vi "Test Path 1.vi"() -> (4 "path":cluster{"X":dbl, "Y":dbl}[](array[cluster])=[{"X"=67.5, "Y"=162.0}, {"X"=149.75257731958763, "Y"=161.43554006968643}, {"X"=169.7938144329897, "Y"=66.60627177700349}, {"X"=262.2061855670103, "Y"=62.09059233449478}, {"X"=279.4639175257732, "Y"=97.65156794425087}, {"X"=279.4639175257732, "Y"=115.14982578397213}])   [LabVIEW 2018]
uses:
  AutonBuilder/Typedef/Data Point.ctl
panel:
  in  "Data Points":T1[](array[typedef])=[{"X"=67.5, "Y"=162.0, "Theta"=0.0, "Speed %"=0.0, "Disabled?"=FALSE}, {"X"=149.75257731958763, "Y"=161.43554006968643, "Theta"=0.0, "Speed %"=0.0, "Disabled?"=FALSE}, {"X"=169.7938144329897, "Y"=66.60627177700349, "Theta"=0.0, "Speed %"=0.0, "Disabled?"=FALSE}, {"X"=262.2061855670103, "Y"=62.09059233449478, "Theta"=0.0, "Speed %"=0.0, "Disabled?"=FALSE}, {"X"=279.4639175257732, "Y"=97.65156794425087, "Theta"=0.0, "Speed %"=0.0, "Disabled?"=FALSE}, {"X"=279.4639175257732, "Y"=115.14982578397213, "Theta"=0.0, "Speed %"=0.0, "Disabled?"=FALSE}]
  out "Graph":cluster{dbl[], dbl[]}[](graph)=[{[48.0, 81.5, 81.5, 48.0, 48.0], [176.25, 176.25, 147.75, 147.75, 176.25]}, {[67.5, 149.75257731958763, 169.7938144329897, 262.2061855670103, 279.4639175257732, 279.4639175257732], [162.0, 161.43554006968643, 66.60627177700349, 62.09059233449478, 97.65156794425087, 115.14982578397213]}, {array[332 elements], array[332 elements]}, {array[332 elements], array[332 elements]}, {array[332 elements], array[332 elements]}]
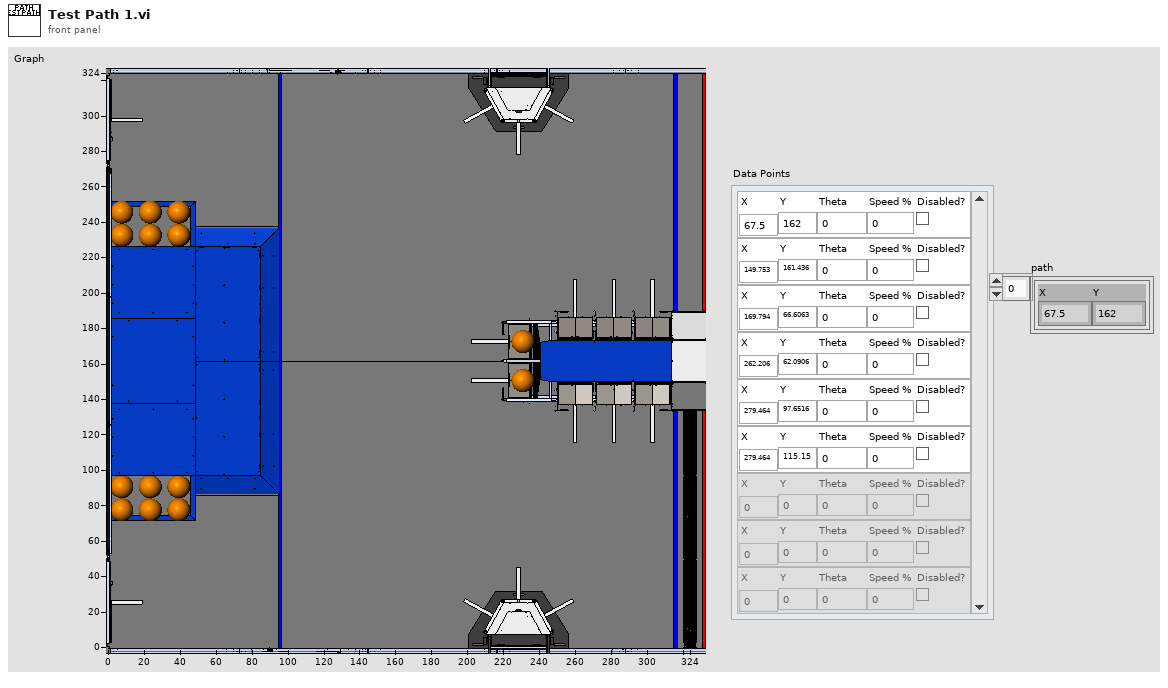
[diagram p1: front panel]
types:
  T1 = typedef "Data Point.ctl" = cluster{"X":dbl, "Y":dbl, "Theta":dbl, "Speed %":dbl, "Disabled?":bool}
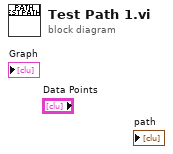
[diagram p0: block diagram]
diagram:
